vi "ALR select.vi"(10 "System":i32, 11 "ALR_State":T2) -> (1 "ALRs":bool[](array[boolean]), 2 "code":i32[](array[numeric]), 3 "ALR_Status":T1[](array[typedef]))   [LabVIEW 2019, in "Alarms.lvlib"]
uses:
  Alarms.lvlib
  Ctl/ALRs_State.ctl
  Ctl/ALR_Status_short.ctl
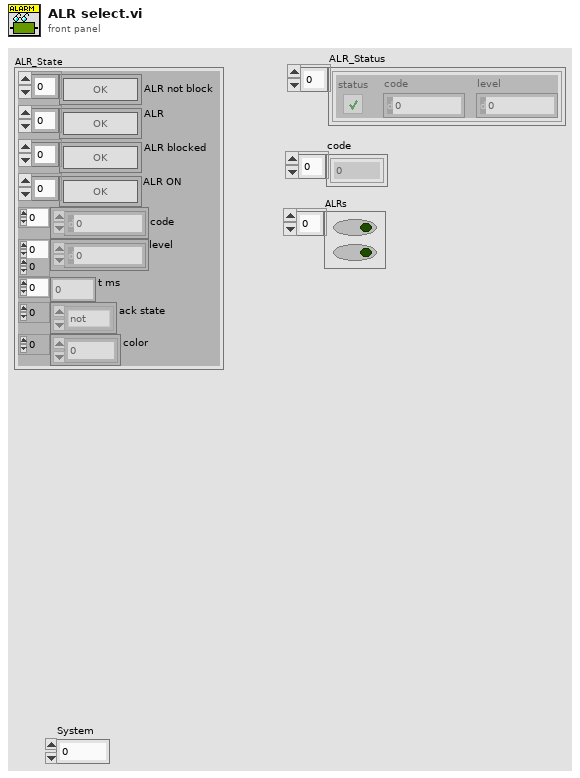
[diagram p1: front panel]
types:
  T1 = typedef "Alarms.lvlib/ALR_Status_short.ctl" = cluster{"status":bool, "code":i32, "level":i32}
  T2 = typedef "Alarms.lvlib/ALRs_State.ctl" = cluster{"ALR not block":bool[], "ALR":bool[], "ALR blocked":bool[], "ALR ON":bool[], "code":i32[], "level":i32[][], "t ms":u32[], "ack state":enum32{"not", "tripped", "reset", "ack"}[], "color":u32[]}
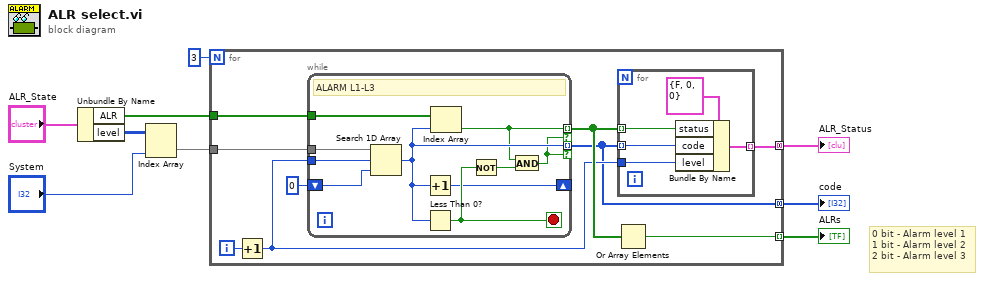
[diagram p0: block diagram]
diagram:
  # "0 bit - Alarm level 1\n1 bit - Alarm level 2\n2 bit - Alarm level 3"
  n1 = Unbundle By Name("ALR_State") -> ("ALR"=w6:bool[], "level"=w8:i32[][])
  n2 = Index Array(array=w8, index (col)="System") -> (element=w5:i32[])  [unwired: 1 in]
  n3 = for {
    N: 3 -> [_]
    tunnel: w6 -> [w17]
    tunnel: w5 -> [w16]
    tunnel: [w11] -> w3 mode=concatenating
    tunnel: [w12] -> w2 mode=indexing
    tunnel: [w10] -> w1 mode=concatenating
    i -> [w15]
    n4 = Increment(x=w15) -> (x+1=w13:i32)
    n5 = while {
      tunnel: w16 -> [w28]
      shift-right: [w22] -> _
      shift-left: 0 ("index of element") -> [w27]
      tunnel: [w24] -> w10 mode=indexing if=w20
      tunnel: w17 -> [w25]
      tunnel: [w19] -> w14 mode=indexing if=w20
      tunnel: w13 -> [w23]
      stop <- w26 stop-if-true
      # "ALARM L1-L3"
      n6 = Search 1D Array(1D array=w28, element=w23, start index (0)=w27) -> (index of element=w24:i32)
      n7 = Increment(x=w24) -> (x+1=w22:i32)
      n8 = Less Than 0?(x=w24) -> (x < 0?=w26:bool)
      n9 = Index Array(array=w25, index=w24) -> (element=w19:bool)
      n10 = Not(x=w26) -> (.not. x?=w21:bool)
      n11 = And(x=w19, y=w21) -> (x .and. y?=w20:bool)
    }
    n12 = for {
      tunnel: w14 -> [w32] mode=indexing
      tunnel: w10 -> [w31] mode=indexing
      tunnel: [w30] -> w11 mode=indexing
      tunnel: w13 -> [w29]
      n13 = Bundle By Name(cluster=T1 {"status"=FALSE, "code"=0, "level"=0} ("ALR_Status"), "status"=w32, "code"=w31, "level"=w29) -> (w30:T1)
    }
    n14 = Or Array Elements(Boolean array=w14) -> (logical OR=w12:bool)
  }
  "ALRs" <- w2
  "ALR_Status" <- w3
  "code" <- w1
